vi "UDT_admittanceLibrary_newTarget2.vi"() -> (3 "Unit Test Framework Results":T1)   [LabVIEW 2017]
doc: "Use this template to create a user-defined test VI. Define your test requirements and wire the results to the <b>Result (Test)</b> control. Do not modify the <b>Unit Test Framework Results</b> indicator."
uses:
  <vilib>/utf/common/utf_test_result_troll.ctl
  <vilib>/utf/common/utf_test_result.ctl
  <vilib>/utf/common/utf_test_result_failure.ctl
  <vilib>/utf/common/utf_test_comparison_operators.ctl
  <vilib>/utf/common/utf_vi_tag.ctl
  <vilib>/Control Software Solutions Ltd/UTF Helper/SubVIs/UTF Boolean Equals.vi
  RT/Admittance Controller/admittanceControllerLibrary.lvlib
  <vilib>/Control Software Solutions Ltd/UTF Helper/Unit Test Helper.lvlib
  <vilib>/utf/NI_UnitTestFramework.lvlib
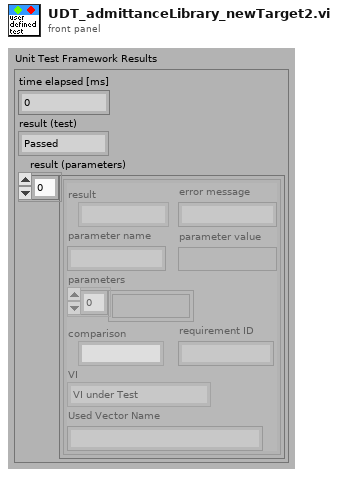
[diagram p1: front panel]
types:
  T1 = typedef "NI_UnitTestFramework.lvlib/utf_test_result_troll.ctl" = cluster{"time elapsed [ms]":u32, "result (test)":T2, "result (parameters)":T3[]}
  T2 = typedef "NI_UnitTestFramework.lvlib/utf_test_result.ctl" = enum16{"Passed", "Failed", "Error", "Skipped", "Not Processed"}
  T3 = typedef "NI_UnitTestFramework.lvlib/utf_test_result_failure.ctl" = cluster{"result":T2, "error message":string, "parameter name":string, "parameter value":variant, "parameters":variant[], "comparison":T4, "requirement ID":string, "VI":T5, "Used Vector Name":string}
  T4 = typedef "NI_UnitTestFramework.lvlib/utf_test_comparison_operators.ctl" = enum16{"=", "!=", ">", ">=", "<", "<=", "range", "symmetric tolerance", "asymmetric tolerance", "string contains", "string not contain", "array size", "string length", "array range", "by element", "array range (limit array)", "user-defined", "array contains", "array not contain", "vector length", "= (elm)", "!= (elm)", "= (case insensitive)", "!= (case insensitive)"}
  T5 = typedef "NI_UnitTestFramework.lvlib/utf_vi_tag.ctl" = enum16{"Setup VI", "VI under Test", "Teardown VI"}
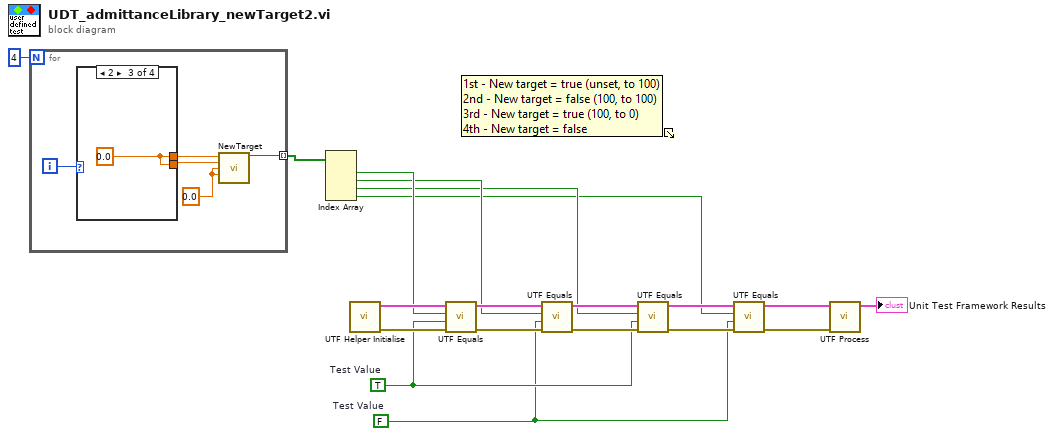
[diagram p0: block diagram]
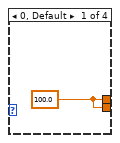
[diagram p2: hidden frame]
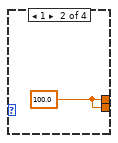
[diagram p3: hidden frame]
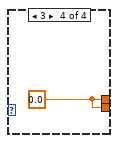
[diagram p4: hidden frame]
diagram:
  w2 = FALSE  # Test Value
  w3 = TRUE  # Test Value
  n1 = for {
    N: 4 -> [_]
    tunnel: [w20] -> w18 mode=indexing
    i -> [w24]
    w23 = 0.0
    n2 = case shown="2" w24 {
      tunnel: [w25 w26 w27 w28] -> w22
      tunnel: [w25 w26 w27 w28] -> w21
      frame 0, Default {
        w25 = 100.0
      }
      frame 1 {
        w26 = 100.0
      }
      frame 2 {
        w27 = 0.0
      }
      frame 3 {
        w28 = 0.0
      }
    }
    n3 = call "NewTarget.vi"("Target x"=w22, "Target y"=w21, "Current x"=w23, "Current y"=w23) -> ("NewTarget"=w20:bool)  [unwired: 10 in, 1 out]
  }
  n4 = Index Array(array=w18) -> (element #1=w7:bool, element #2=w6:bool, element #3=w5:bool, element #4=w4:bool)  [unwired: 4 in]
  n5 = call <vilib>:"UTF Helper Initialise.vi"() -> ("error out"=w17:errorcluster, "results array"=w16:T3[])  [unwired: 10 in]
  n6 = call-poly <vilib>:"UTF Equals.vi"("error in (no error)"=w17, "Test Value"=w3, "Input"=w7, "Input Results"=w16) -> ("error out"=w8:errorcluster, "Output Results"=w15:T3[])  [unwired: 6 in]
  n7 = call-poly <vilib>:"UTF Equals.vi"("error in (no error)"=w8, "Test Value"=w2, "Input"=w6, "Input Results"=w15) -> ("error out"=w9:errorcluster, "Output Results"=w14:T3[])  [unwired: 6 in]
  n8 = call-poly <vilib>:"UTF Equals.vi"("error in (no error)"=w9, "Test Value"=w3, "Input"=w5, "Input Results"=w14) -> ("error out"=w10:errorcluster, "Output Results"=w13:T3[])  [unwired: 6 in]
  n9 = call-poly <vilib>:"UTF Equals.vi"("error in (no error)"=w10, "Test Value"=w2, "Input"=w4, "Input Results"=w13) -> ("error out"=w11:errorcluster, "Output Results"=w12:T3[])  [unwired: 6 in]
  n10 = call <vilib>:"UTF Process.vi"("error in (no error)"=w11, "results array"=w12) -> ("Unit Test Framework Results"=→"Unit Test Framework Results":T1)  [unwired: 9 in]
